vi "PixmapToFXP.vi"(11 "image data in":T1) -> (2 "FXPdata":fxp<+,3,3>[](array[numeric]), 3 "image data out":T1)   [LabVIEW 2019, in "Initializers.lvlib"]
uses:
  Initializers.lvlib
  <vilib>/picture/picture.llb/imagedata.ctl
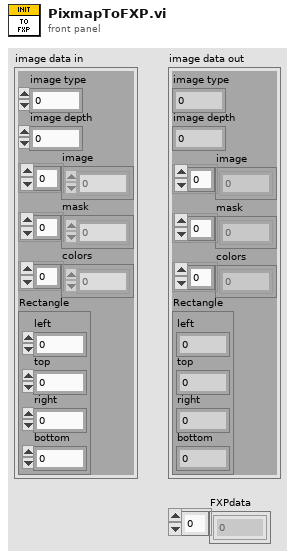
[diagram p1: front panel]
types:
  T1 = typedef "imagedata.ctl" = cluster{"image type":i32, "image depth":i32, "image":u8[], "mask":u8[], "colors":u32[], "Rectangle":cluster{"left":i16, "top":i16, "right":i16, "bottom":i16}}
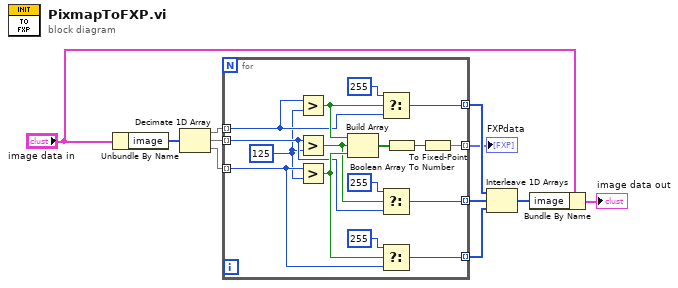
[diagram p0: block diagram]
diagram:
  n1 = Unbundle By Name("image data in") -> ("image"=w7:u8[])
  n2 = Decimate 1D Array(w7) -> (w8:u8[], w9:u8[], w10:u8[])
  n3 = for {
    tunnel: w8 -> [w16] mode=indexing
    tunnel: w9 -> [w20] mode=indexing
    tunnel: w10 -> [w19] mode=indexing
    tunnel: [w25] -> w1 mode=indexing
    tunnel: [w14] -> w4 mode=indexing
    tunnel: [w13] -> w3 mode=indexing
    tunnel: [w12] -> w2 mode=indexing
    w15 = u8 125 ("y")
    n4 = Greater?(x=w16, y=w15) -> (0:w24:bool)
    n5 = Greater?(x=w20, y=w15) -> (0:w22:bool)
    n6 = Greater?(x=w19, y=w15) -> (0:w23:bool)
    n7 = Build Array(w24, w22, w23) -> (w27:bool[])
    n8 = Select(t=u8 255, s=w24, f=w16) -> (s? t:f=w14:u8)
    n9 = Select(t=u8 255, s=w22, f=w20) -> (s? t:f=w13:u8)
    n10 = Select(t=u8 255, s=w23, f=w19) -> (s? t:f=w12:u8)
    n11 = Boolean Array To Number(Boolean array=w27) -> (number=w26:u32)
    n12 = To Fixed-Point(number=w26) -> (fixed-point=w25:fxp<+,3,3>)  [unwired: 1 in]
  }
  "FXPdata" <- w1
  n13 = Interleave 1D Arrays(w4, w3, w2) -> (w6:u8[])
  n14 = Bundle By Name(cluster="image data in", "image"=w6) -> (→"image data out":T1)
